vi "Configure TV Trig Line Number.vi"(8 "error in (no error)":errorcluster {"code" format="%.0x"}, 10 "line count (1)":i32=1 caption="Line Count (1)", 11 "VISA Resource Name":refnum<visa-resource-name>) -> (0 "error out":errorcluster {"code" format="%.0x"}, 3 "VISA Resource Name Out":refnum<visa-resource-name>)   [LabVIEW 2011, in "Agilent 546XX Series.lvlib"]
doc: "This VI configures the line or vertical count on which TV trigger is set.\n\nNotes:\n\n(1) This VI affects instrument behavior only if the Trigger Type is TV Trigger. Call the ag546xx Configure Trigger VI to set the Trigger Type before you call this VI."
uses:
  Agilent 546XX Series.lvlib
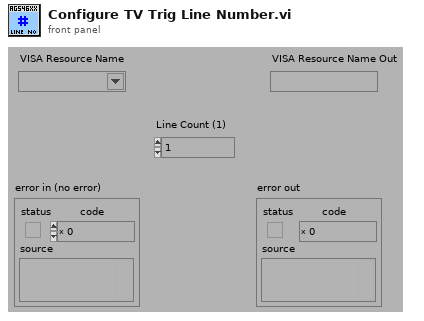
[diagram p1: front panel]
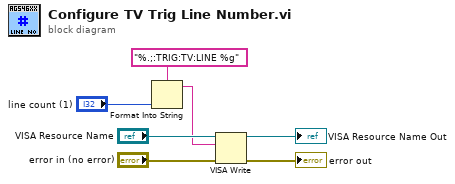
[diagram p0: block diagram]
diagram:
  n1 = Format Into String(format string="%.;:TRIG:TV:LINE %g", "line count (1)") -> (resulting string=w1:string)  [unwired: 2 in, 1 out]
  n2 = VISA Write(VISA resource name="VISA Resource Name", write buffer=w1, error in (no error)="error in (no error)") -> (VISA resource name out=→"VISA Resource Name Out":refnum<visa-resource-name>, error out=→"error out":errorcluster)  [unwired: 1 out]
